vi "init.vi"() -> ()   [LabVIEW 2013]
uses:
  <vilib>/Instr/_visa.llb/VISA Configure Serial Port (Instr).vi
panel:
  out "error out":errorcluster
  out "VISA resource name out":refnum<visa-resource-name>
  in  "error in (no error)":errorcluster
  in  "VISA resource name":refnum<visa-resource-name>
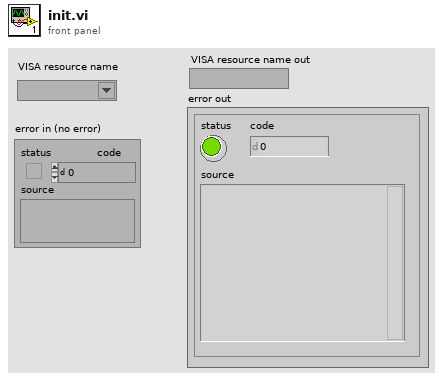
[diagram p1: front panel]
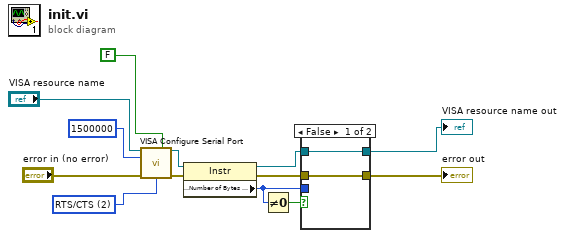
[diagram p0: block diagram]
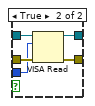
[diagram p2: hidden frame]
diagram:
  w1 = u16 2 items=["None", "XON/XOFF", "RTS/CTS", "XON/XOFF & RTS/CTS", "DTR/DSR", "XON/XOFF & DTR/DSR"] ("flow control (0:none)")
  n1 = call-poly "VISA Configure Serial Port"("VISA resource name"="VISA resource name", "Enable Termination\nChar (T)"=FALSE ("Enable Termination\nChar (T)"), "baud rate (9600)"=u32 1500000, "error in (no error)"="error in (no error)", "flow control (0:none)"=w1) -> ("VISA resource name out"=w8:refnum<visa-resource-name>, "error out"=w9:errorcluster)  [unwired: 9 in]
  n2 = property class="Instr"(reference=w8, error in=w9) -> (reference out=w7:refnum<visa-resource-name>, error out=w6:errorcluster, "Serial Settings:Number of Bytes at Serial Port"=w4:u32)
  n3 = Not Equal To 0?(x=w4) -> (x != 0?=w5:bool)
  n4 = case shown="False" w5 {
    tunnel: w7 -> [w15 w20]
    tunnel: w6 -> [w14 w19]
    tunnel: w4 -> [_ w18]
    tunnel: [w15 w17] -> w3
    tunnel: [w14 w16] -> w2
    frame False {
    }
    frame True {
      n5 = VISA Read(VISA resource name=w20, byte count=w18, error in (no error)=w19) -> (VISA resource name out=w17:refnum<visa-resource-name>, error out=w16:errorcluster)  [unwired: 2 out]
    }
  }
  "VISA resource name out" <- w3
  "error out" <- w2
